vi "Convert Unit (CDB).vi"(4 "Quantity":T1, 5 "error in (no error)":errorcluster, 6 "Target Unit":T2, 7 "Base Unit":T2, 8 "Data":cdb) -> (0 "error out":errorcluster, 3 "Converted Data":cdb)   [LabVIEW 2023, in "NI_HFNetworkAnalysis.lvlib"]
doc: "Convert data for a specified quantity from a base unit to a new unit."
uses:
  NI_HFNetworkAnalysis.lvlib
  Controls/Unit.ctl
  Controls/Quantity.ctl
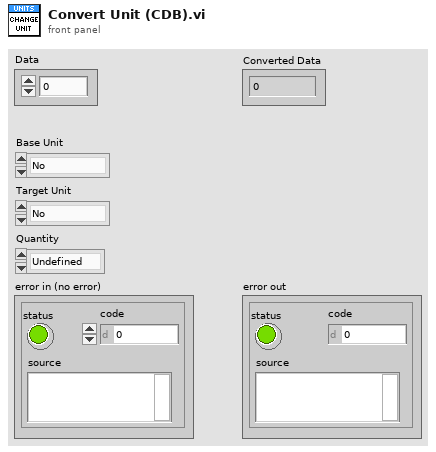
[diagram p1: front panel]
types:
  T1 = typedef "NI_HFNetworkAnalysis.lvlib/Quantity.ctl" = enum16{"Undefined", "V", "I", "A", "B", "P", "Z", "PowerRatio", "Gamma", "Index"}
  T2 = typedef "NI_HFNetworkAnalysis.lvlib/Unit.ctl" = enum16{"No", "s", "Hz", "V", "A", "Ohm", "W", "dB", "dBV", "dBA", "dBm", "percent", "rad", "deg"}
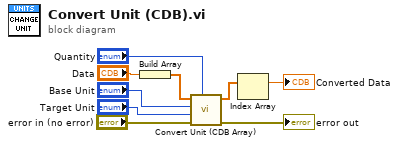
[diagram p0: block diagram]
diagram:
  n1 = Build Array("Data") -> (w3:cdb[])
  n2 = call "Convert Unit (CDB Array).vi"("Quantity"="Quantity", "error in (no error)"="error in (no error)", "Target Unit"="Target Unit", "Base Unit"="Base Unit", "Data"=w3) -> ("error out"=→"error out":errorcluster, "Converted Data"=w2:cdb[])  [unwired: 2 in]
  n3 = Index Array(array=w2) -> (element=→"Converted Data":cdb)  [unwired: 1 in]
